vi "Set TC Parameters.vi"() -> ()   [LabVIEW 2020]
uses:
  _libraries/Startup Processes/_typedefs/Subpanel Names.ctl
  _libraries/Startup Processes/_typedefs/TC Setup Parameters.ctl
  toolbox/Standard Signalling/not_Generic Named Notifier/not_Generic Named Notifier.lvlib
  _ude/Set TC Parameters/Set TC Parameters.lvlib
  _libraries/Startup Processes/Startup Processes.lvlib
panel:
  out "Raw Response":variant
  out "Error Out":errorcluster
  in  "TC Parameters":T1
  in  "Plugin Names":T2
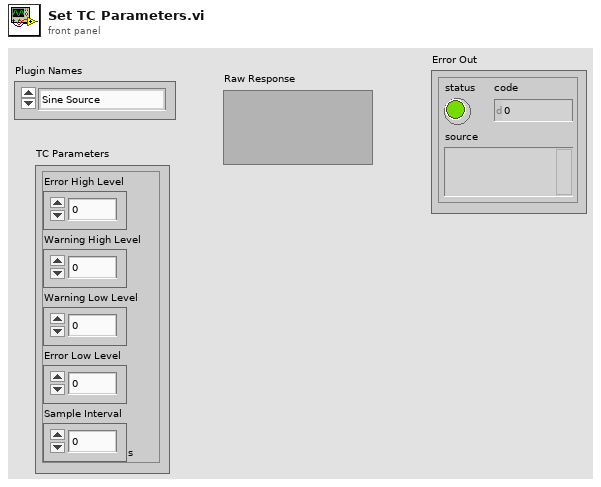
[diagram p1: front panel]
types:
  T1 = typedef "Startup Processes.lvlib/TC Setup Parameters.ctl" = cluster{"Error High Level":dbl, "Warning High Level":dbl, "Warning Low Level":dbl, "Error Low Level":dbl, "Sample Interval":dbl[unit]}
  T2 = typedef "Startup Processes.lvlib/Subpanel Names.ctl" = enum16{"Sine Source", "Ramp Source", "Hen House TC", "Dog House TC", "Out House TC"}
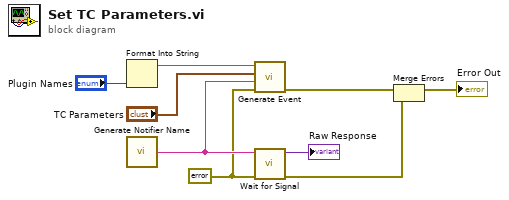
[diagram p0: block diagram]
diagram:
  w2 = errorcluster {"status"=FALSE, "code"=0, "source"=""} ("Error In")
  n1 = Format Into String("Plugin Names") -> (resulting string=w5:string)  [unwired: 3 in, 1 out]
  n2 = call "Generate Notifier Name.vi"() -> ("Notifier Name"=w4:string)
  n3 = call "Generate Event.vi"("Error In"=w2, "Response Notifier"=w4, "TC Parameters"="TC Parameters", "Plugin Name"=w5) -> ("Error Out"=w3:errorcluster)  [unwired: 3 in]
  n4 = call "Wait for Signal.vi"("Error In"=w2, "Notifier Name"=w4) -> ("Error Out"=w6:errorcluster, "Signal Data"=→"Raw Response":variant)  [unwired: 4 in]
  n5 = Merge Errors(w3, w6) -> (→"Error Out":errorcluster)
